vi "CD Config Settings FG.vi"(6 "Action":T2, 7 "UI Refs":T1, 8 "error in (no error)":errorcluster, 10 "CD Settings in":T3={"CD Task Dependency"=18446744073709551615, "CD Task Dependency Ref"=18446744073709551615, "CD Task Available Wfms"=[], "CD Task Selected Wfms"=[], "Buffer Length (s)"=0.0, "Buffer Length (samples)"=0, "Single-point Enabled"=FALSE, "Running Average Enabled"=FALSE, "Task Rate"=0.0, "Scaled Waveform Enabled"=FALSE} {"CD Task Dependency Ref" format="%.0x"; "CD Task Dependency" format="%.0x"}, 11 "Item Ref":T4 format="%.0x") -> (0 "error out":errorcluster, 2 "CD Settings out":T3={"CD Task Dependency"=18446744073709551615, "CD Task Dependency Ref"=18446744073709551615, "CD Task Available Wfms"=[], "CD Task Selected Wfms"=[], "Buffer Length (s)"=0.0, "Buffer Length (samples)"=0, "Single-point Enabled"=FALSE, "Running Average Enabled"=FALSE, "Task Rate"=0.0, "Scaled Waveform Enabled"=FALSE} {"CD Task Dependency Ref" format="%.0x"; "CD Task Dependency" format="%.0x"}, 3 "Item Ref out":T4=18446744073709551615 format="%.0x", 5 "UI Refs out":T1)   [LabVIEW 2020, in "Waveform-Processing-Custom-Device Shared.lvlib"]
uses:
  Waveform-Processing-Custom-Device Shared.lvlib
  <vilib>/NI VeriStand/Custom Device API/Custom Device Item Ref.ctl
  Custom Device Settings.ctl
  Types/FG Action.ctl
  System Explorer/Types/UI Refs Ctl.ctl
  Constants.vi
  <vilib>/NI VeriStand/Custom Device API/Get Item Property (Dependent Node Pointer).vi
  <vilib>/NI VeriStand/Custom Device API/Get Item Property (String Array).vi
  <vilib>/NI VeriStand/Custom Device API/Get Item Property (Double).vi
  <vilib>/NI VeriStand/Custom Device API/Get Item Property (U32).vi
  <vilib>/NI VeriStand/Custom Device API/Get Item Property (Boolean).vi
  <vilib>/NI VeriStand/Custom Device API/Set Item Property (Dependent Node Pointer).vi
  <vilib>/NI VeriStand/Custom Device API/Set Item Property (String Array).vi
  <vilib>/NI VeriStand/Custom Device API/Set Item Property (U32).vi
  <vilib>/NI VeriStand/Custom Device API/Set Item Property (Boolean).vi
  <vilib>/NI VeriStand/Custom Device API/Set Item Property (Double).vi
  <vilib>/NI VeriStand/Custom Device API/Custom Device API.lvlib
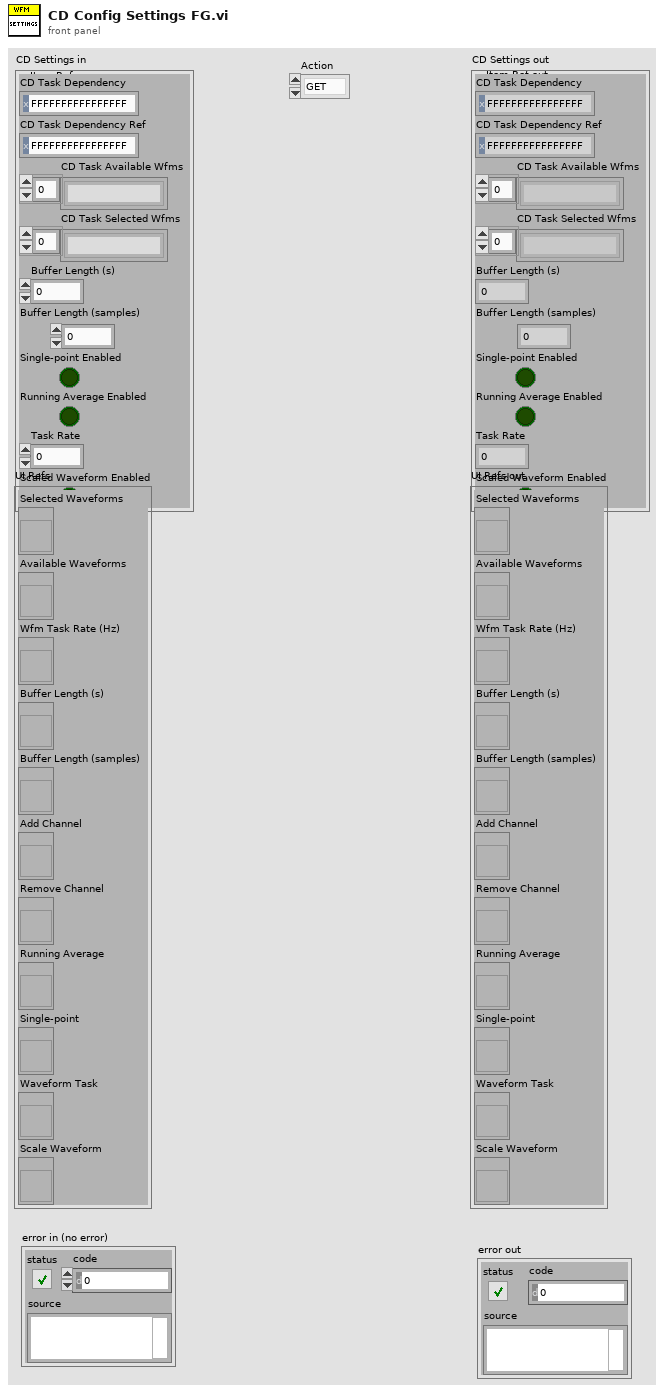
[diagram p1: front panel]
types:
  T1 = typedef "Waveform-Processing-Custom-Device Shared.lvlib/UI Refs Ctl.ctl" = cluster{"Selected Waveforms":refnum<vi>, "Available Waveforms":refnum<vi>, "Wfm Task Rate (Hz)":refnum<vi>, "Buffer Length (s)":refnum<vi>, "Buffer Length (samples)":refnum<vi>, "Add Channel":refnum<vi>, "Remove Channel":refnum<vi>, "Running Average":refnum<vi>, "Single-point":refnum<vi>, "Waveform Task":refnum<vi>, "Scale Waveform":refnum<vi>}
  T2 = typedef "Waveform-Processing-Custom-Device Shared.lvlib/FG Action.ctl" = enum8{"GET", "SET"}
  T3 = typedef "Waveform-Processing-Custom-Device Shared.lvlib/Custom Device Settings.ctl" = cluster{"CD Task Dependency":T4, "CD Task Dependency Ref":T4, "CD Task Available Wfms":string[], "CD Task Selected Wfms":string[], "Buffer Length (s)":dbl, "Buffer Length (samples)":u32, "Single-point Enabled":bool, "Running Average Enabled":bool, "Task Rate":dbl, "Scaled Waveform Enabled":bool}
  T4 = typedef "Custom Device API.lvlib/Custom Device Item Ref.ctl" = u64
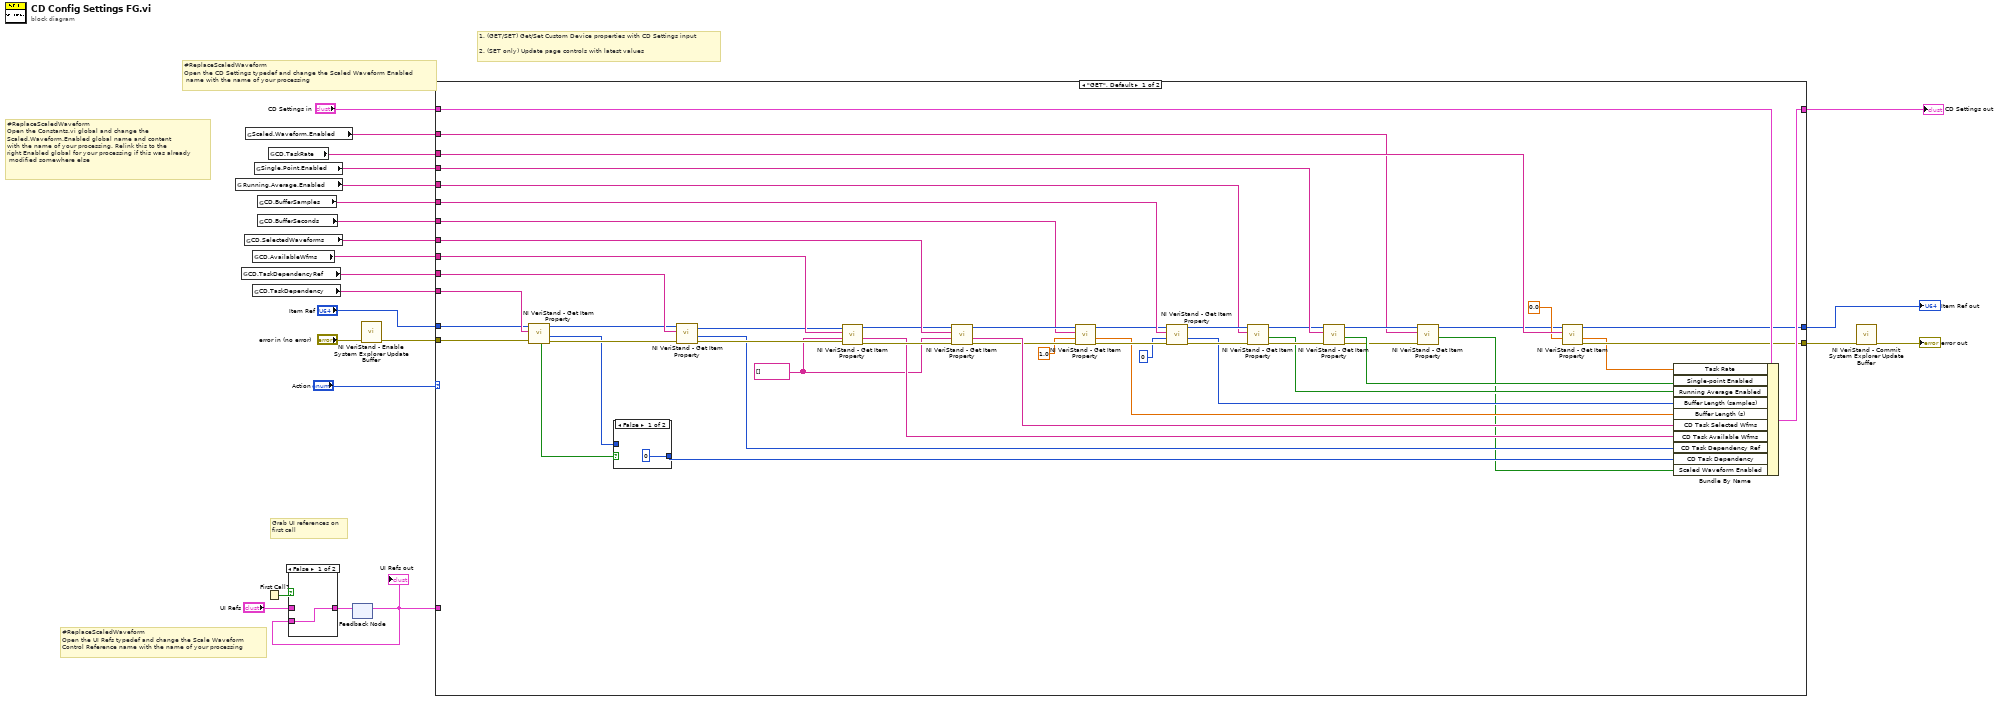
[diagram p0: block diagram]
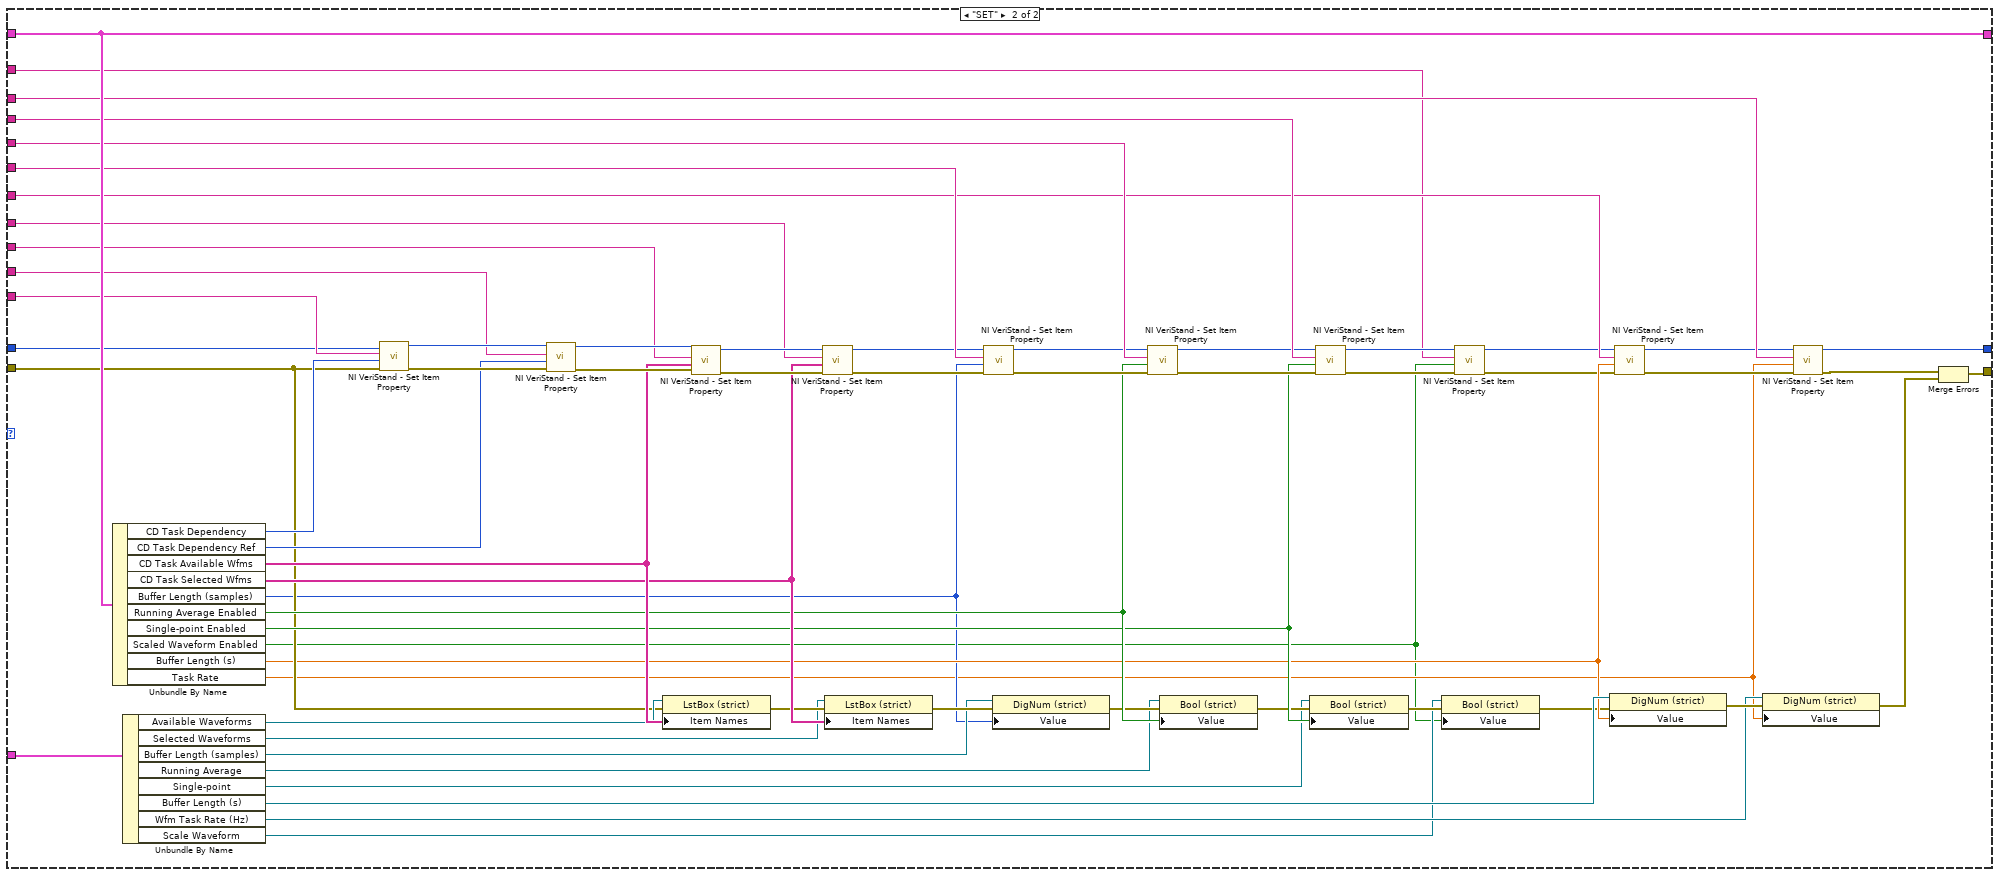
[diagram p4: hidden frame]
diagram:
  # "#ReplaceScaledWaveform \nOpen the Constants.vi global and change the \nScaled.Waveform.Enabled global name and content \nwith the name of your processing. Relink this to the \nright Enabled global for your processing if this was already\n modified somewhere else"
  # "#ReplaceScaledWaveform \nOpen the CD Settings typedef and change the Scaled Waveform Enabled\n name with the name of your processing"
  # "#ReplaceScaledWaveform \nOpen the UI Refs typedef and change the Scale Waveform\nControl Reference name with the name of your processing"
  # "Grab UI references on\nfirst call"
  # "1. (GET/SET) Get/Set Custom Device properties with CD Settings input\n\n2. (SET only) Update page controls with latest values"
  n1 = global read "Constants.vi" "Running.Average.Enabled"() -> (w19:string)
  n2 = global read "Constants.vi" "CD.TaskDependencyRef"() -> (w22:string)
  n3 = global read "Constants.vi" "CD.SelectedWaveforms"() -> (w20:string)
  n4 = global read "Constants.vi" "Scaled.Waveform.Enabled"() -> (w1:string)
  n5 = global read "Constants.vi" "CD.AvailableWfms"() -> (w21:string)
  n6 = global read "Constants.vi" "CD.TaskDependency"() -> (w23:string)
  n7 = global read "Constants.vi" "Single.Point.Enabled"() -> (w18:string)
  n8 = global read "Constants.vi" "CD.BufferSamples"() -> (w4:string)
  n9 = global read "Constants.vi" "CD.BufferSeconds"() -> (w3:string)
  n10 = First Call?() -> (First Call?: T/F=w8:bool)
  n11 = global read "Constants.vi" "CD.TaskRate"() -> (w2:string)
  n12 = feedback #1() -> (w5:T1)  [unwired: 1 in]
  "UI Refs out" <- w5
  n13 = case shown="False" w8 {
    tunnel: "UI Refs" -> [_ w25]
    tunnel: [w24 w25] -> w7
    tunnel: w5 -> [w24 _]
    frame False {
    }
    frame True {
    }
  }
  n14 = feedback-in #1(w7) -> ()
  n15 = call <vilib>:"NI VeriStand - Enable System Explorer Update Buffer.vi"("error in (no error)"="error in (no error)") -> ("error out"=w13:errorcluster)  [unwired: 10 in]
  n16 = case shown="\"GET\", Default" "Action" {
    tunnel: w13 -> [w74 w101]
    tunnel: "Item Ref" -> [w72 w134]
    tunnel: "CD Settings in" -> [w55 w137]
    tunnel: w23 -> [w73 w135]
    tunnel: w22 -> [w70 w132]
    tunnel: w21 -> [w68 w129]
    tunnel: w20 -> [w64 w126]
    tunnel: w4 -> [w62 w124]
    tunnel: w19 -> [w59 w121]
    tunnel: w18 -> [w57 w119]
    tunnel: [w35 w100] -> w10
    tunnel: [w34 w91] -> w11
    tunnel: [w47 w137] -> w17
    tunnel: w5 -> [_ w99]
    tunnel: w3 -> [w39 w97]
    tunnel: w2 -> [w33 w94]
    tunnel: w1 -> [w26 w81]
    frame "GET", Default {
      w52 = string[] [] ("Default Value")
      n17 = call-poly <vilib>:"NI VeriStand - Get Item Property.vi"("error in (no error)"=w74, "Property Name"=w73, "Item Ref in"=w72) -> ("error out"=w71:errorcluster, "Dependent Node Ref"=w45:T4, "Item Ref out"=w69:T4, "Found"=w46:bool)  [unwired: 5 in]
      n18 = case shown="False" w46 {
        tunnel: w45 -> [_ w76]
        tunnel: [T4 0 ("Dependent Node Ref") w76] -> w44
        frame False {
        }
        frame True {
        }
      }
      n19 = call-poly <vilib>:"NI VeriStand - Get Item Property.vi"("error in (no error)"=w71, "Property Name"=w70, "Item Ref in"=w69) -> ("error out"=w67:errorcluster, "Dependent Node Ref"=w54:T4, "Item Ref out"=w65:T4)  [unwired: 5 in, 1 out]
      n20 = call-poly <vilib>:"NI VeriStand - Get Item Property.vi"("error in (no error)"=w67, "Default Value"=w52, "Property Name"=w68, "Item Ref in"=w65) -> ("error out"=w66:errorcluster, "Value"=w53:string[], "Item Ref out"=w63:T4)  [unwired: 4 in, 1 out]
      n21 = call-poly <vilib>:"NI VeriStand - Get Item Property.vi"("error in (no error)"=w66, "Default Value"=w52, "Property Name"=w64, "Item Ref in"=w63) -> ("error out"=w43:errorcluster, "Value"=w51:string[], "Item Ref out"=w42:T4)  [unwired: 4 in, 1 out]
      n22 = call-poly <vilib>:"NI VeriStand - Get Item Property.vi"("error in (no error)"=w43, "Default Value"=1.0, "Property Name"=w39, "Item Ref in"=w42) -> ("error out"=w40:errorcluster, "Value"=w37:dbl, "Item Ref out"=w41:T4)  [unwired: 4 in, 1 out]
      n23 = call-poly <vilib>:"NI VeriStand - Get Item Property.vi"("error in (no error)"=w40, "Default Value"=u32 0, "Property Name"=w62, "Item Ref in"=w41) -> ("error out"=w61:errorcluster, "Value"=w50:u32, "Item Ref out"=w60:T4)  [unwired: 4 in, 1 out]
      n24 = call-poly <vilib>:"NI VeriStand - Get Item Property.vi"("error in (no error)"=w61, "Property Name"=w59, "Item Ref in"=w60) -> ("error out"=w58:errorcluster, "Value"=w49:bool, "Item Ref out"=w56:T4)  [unwired: 5 in, 1 out]
      n25 = call-poly <vilib>:"NI VeriStand - Get Item Property.vi"("error in (no error)"=w58, "Property Name"=w57, "Item Ref in"=w56) -> ("error out"=w30:errorcluster, "Value"=w48:bool, "Item Ref out"=w29:T4)  [unwired: 5 in, 1 out]
      n26 = call-poly <vilib>:"NI VeriStand - Get Item Property.vi"("error in (no error)"=w30, "Property Name"=w26, "Item Ref in"=w29) -> ("Value"=w27:bool, "Item Ref out"=w28:T4)  [unwired: 5 in, 2 out]
      n27 = call-poly <vilib>:"NI VeriStand - Get Item Property.vi"("Default Value"=0.0, "Property Name"=w33, "Item Ref in"=w28) -> ("error out"=w35:errorcluster, "Value"=w31:dbl, "Item Ref out"=w34:T4)  [unwired: 5 in, 1 out]
      n28 = Bundle By Name(cluster=w55, "Task Rate"=w31, "Single-point Enabled"=w48, "Running Average Enabled"=w49, "Buffer Length (samples)"=w50, "Buffer Length (s)"=w37, "CD Task Selected Wfms"=w51, "CD Task Available Wfms"=w53, "CD Task Dependency Ref"=w54, "CD Task Dependency"=w44, "Scaled Waveform Enabled"=w27) -> (w47:T3)
    }
    frame "SET" {
      n29 = Unbundle By Name(w137) -> ("CD Task Dependency"=w116:T4, "CD Task Dependency Ref"=w115:T4, "CD Task Available Wfms"=w114:string[], "CD Task Selected Wfms"=w113:string[], "Buffer Length (samples)"=w95:u32, "Running Average Enabled"=w110:bool, "Single-point Enabled"=w108:bool, "Scaled Waveform Enabled"=w77:bool, "Buffer Length (s)"=w96:dbl, "Task Rate"=w87:dbl)
      n30 = Unbundle By Name(w99) -> ("Available Waveforms"=w102:refnum<vi>, "Selected Waveforms"=w103:refnum<vi>, "Buffer Length (samples)"=w104:refnum<vi>, "Running Average"=w105:refnum<vi>, "Single-point"=w106:refnum<vi>, "Buffer Length (s)"=w98:refnum<vi>, "Wfm Task Rate (Hz)"=w88:refnum<vi>, "Scale Waveform"=w78:refnum<vi>)
      n31 = call-poly <vilib>:"NI VeriStand - Set Item Property.vi"("error in (no error)"=w101, "Dependent Node Ref"=w116, "Property Name"=w135, "Item Ref in"=w134) -> ("error out"=w136:errorcluster, "Item Ref out"=w133:T4)  [unwired: 5 in, 1 out]
      n32 = call-poly <vilib>:"NI VeriStand - Set Item Property.vi"("error in (no error)"=w136, "Dependent Node Ref"=w115, "Property Name"=w132, "Item Ref in"=w133) -> ("error out"=w131:errorcluster, "Item Ref out"=w130:T4)  [unwired: 5 in, 1 out]
      n33 = property class="LstBox (strict)"(reference=w102, error in=w101, "Item Names"=w114) -> (error out=w112:errorcluster)  [unwired: 1 out]
      n34 = call-poly <vilib>:"NI VeriStand - Set Item Property.vi"("error in (no error)"=w131, "Value"=w114, "Property Name"=w129, "Item Ref in"=w130) -> ("error out"=w128:errorcluster, "Item Ref out"=w127:T4)  [unwired: 5 in, 1 out]
      n35 = call-poly <vilib>:"NI VeriStand - Set Item Property.vi"("error in (no error)"=w128, "Value"=w113, "Property Name"=w126, "Item Ref in"=w127) -> ("error out"=w125:errorcluster, "Item Ref out"=w123:T4)  [unwired: 5 in, 1 out]
      n36 = property class="LstBox (strict)"(reference=w103, error in=w112, "Item Names"=w113) -> (error out=w111:errorcluster)  [unwired: 1 out]
      n37 = call-poly <vilib>:"NI VeriStand - Set Item Property.vi"("error in (no error)"=w125, "Value"=w95, "Property Name"=w124, "Item Ref in"=w123) -> ("error out"=w122:errorcluster, "Item Ref out"=w118:T4)  [unwired: 5 in, 1 out]
      n38 = property class="DigNum (strict)"(reference=w104, error in=w111, "Value"=w95) -> (error out=w109:errorcluster)  [unwired: 1 out]
      n39 = call-poly <vilib>:"NI VeriStand - Set Item Property.vi"("error in (no error)"=w122, "Value"=w110, "Property Name"=w121, "Item Ref in"=w118) -> ("error out"=w120:errorcluster, "Item Ref out"=w117:T4)  [unwired: 5 in, 1 out]
      n40 = property class="Bool (strict)"(reference=w105, error in=w109, "Value"=w110) -> (error out=w107:errorcluster)  [unwired: 1 out]
      n41 = property class="Bool (strict)"(reference=w106, error in=w107, "Value"=w108) -> (error out=w80:errorcluster)  [unwired: 1 out]
      n42 = call-poly <vilib>:"NI VeriStand - Set Item Property.vi"("error in (no error)"=w120, "Value"=w108, "Property Name"=w119, "Item Ref in"=w117) -> ("error out"=w83:errorcluster, "Item Ref out"=w85:T4)  [unwired: 5 in, 1 out]
      n43 = property class="Bool (strict)"(reference=w78, error in=w80, "Value"=w77) -> (error out=w79:errorcluster)  [unwired: 1 out]
      n44 = call-poly <vilib>:"NI VeriStand - Set Item Property.vi"("error in (no error)"=w83, "Value"=w77, "Property Name"=w81, "Item Ref in"=w85) -> ("error out"=w82:errorcluster, "Item Ref out"=w84:T4)  [unwired: 5 in, 1 out]
      n45 = property class="DigNum (strict)"(reference=w98, error in=w79, "Value"=w96) -> (error out=w89:errorcluster)  [unwired: 1 out]
      n46 = call-poly <vilib>:"NI VeriStand - Set Item Property.vi"("error in (no error)"=w82, "Value"=w96, "Property Name"=w97, "Item Ref in"=w84) -> ("error out"=w93:errorcluster, "Item Ref out"=w90:T4)  [unwired: 5 in, 1 out]
      n47 = property class="DigNum (strict)"(reference=w88, error in=w89, "Value"=w87) -> (error out=w86:errorcluster)  [unwired: 1 out]
      n48 = call-poly <vilib>:"NI VeriStand - Set Item Property.vi"("error in (no error)"=w93, "Value"=w87, "Property Name"=w94, "Item Ref in"=w90) -> ("error out"=w92:errorcluster, "Item Ref out"=w91:T4)  [unwired: 5 in, 1 out]
      n49 = Merge Errors(w92, w86) -> (w100:errorcluster)
    }
  }
  "Item Ref out" <- w11
  "CD Settings out" <- w17
  n50 = call <vilib>:"NI VeriStand - Commit System Explorer Update Buffer.vi"("error in (no error)"=w10) -> ("error out"=→"error out":errorcluster)  [unwired: 10 in]
